vi "Get Data.vi"(8 "error in":errorcluster, 11 "3022A in":refnum<class "3022A.lvclass">) -> (0 "error out":errorcluster, 2 "DataOut":refnum<class "Data.lvclass">[](array[class]), 3 "3022A out":refnum<class "3022A.lvclass">)   [LabVIEW 2014, in "3022A.lvclass"]
doc: "Send a command to get the concentration. The index will indicate which concentration to retrieve, the default being the FP concentration."
uses:
  3022A.lvclass
  Controls/3022A/Enum Cmd.ctl
  reusable/Data/Array Data/Single 1-D/Single_Array.lvclass
  reusable/Data/Data.lvclass
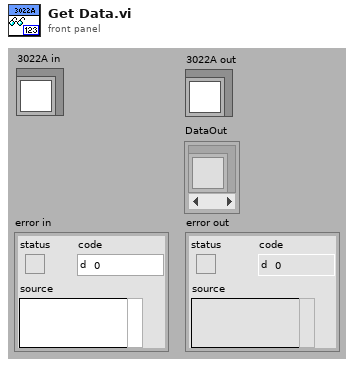
[diagram p1: front panel]
types:
  T1 = typedef "3022A.lvclass/Enum Cmd.ctl" = enum8{"CALIBRATE", "GET CAL DATA", "DUMP", "ESCAPE", "ID CAL LABEL", "INPUT CAL LABEL", "LIQUID LEVEL", "CONDENSER T", "SATURATOR T", "OPTICS T", "GET FLOW RATE", "READ ENV", "READ REF DETECTOR", "READ DETECTOR V", "READ 200 s BUFFER", "READ 20 s BUFFER", "READ 2 s BUFFER", "READ 1 s BUFFER", "READ PHOTOMETRIC CONC", "READ FP CONC", "READ MICROPROCESSOR PUMP CTL", "SENSOR", "SET VOLTAGE", "WRITE DISP MSG", "LASER OFF", "LASER ON", "PUMP OFF", "PUMP ON", "DRAIN", "FILL", "RESET CONC BUFFERS", "LOW FLOW MODE", "HIGH FLOW MODE"}
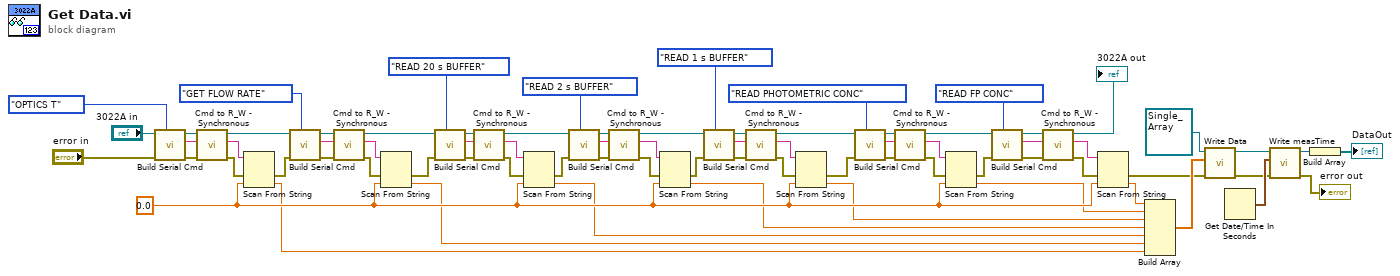
[diagram p0: block diagram]
diagram:
  w8 = sgl 0.0 ("default value 1")
  n1 = call-dynamic "Build Serial Cmd.vi"("Cmd"=Enum_Cmd."OPTICS T", "error in (no error)"="error in", "3022A in"="3022A in") -> ("error out"=w69:errorcluster, "Cmd Out"=w71:string, "3022A out"=w70:refnum<class "3022A.lvclass">)  [unwired: 6 in]
  n2 = call-dynamic "Cmd to R_W - Synchronous.vi"("error in"=w69, "write buffer"=w71, "Serial IO in"=w70) -> ("error out"=w68:errorcluster, "read buffer"=w67:string, "Serial IO out"=w56:refnum<class "3022A.lvclass">)  [unwired: 6 in]
  n3 = Scan From String(input string=w67, error in=w68, default 1=w8) -> (error out=w55:errorcluster, output 1=w7:sgl)  [unwired: 2 in, 2 out]
  n4 = call-dynamic "Build Serial Cmd.vi"("Cmd"=Enum_Cmd."GET FLOW RATE", "error in (no error)"=w55, "3022A in"=w56) -> ("error out"=w60:errorcluster, "Cmd Out"=w58:string, "3022A out"=w59:refnum<class "3022A.lvclass">)  [unwired: 6 in]
  n5 = call-dynamic "Cmd to R_W - Synchronous.vi"("error in"=w60, "write buffer"=w58, "Serial IO in"=w59) -> ("error out"=w61:errorcluster, "read buffer"=w62:string, "Serial IO out"=w42:refnum<class "3022A.lvclass">)  [unwired: 6 in]
  n6 = Scan From String(input string=w62, error in=w61, default 1=w8) -> (error out=w22:errorcluster, output 1=w6:sgl)  [unwired: 2 in, 2 out]
  n7 = call-dynamic "Build Serial Cmd.vi"("Cmd"=Enum_Cmd."READ 20 s BUFFER", "error in (no error)"=w22, "3022A in"=w42) -> ("error out"=w21:errorcluster, "Cmd Out"=w50:string, "3022A out"=w49:refnum<class "3022A.lvclass">)  [unwired: 6 in]
  n8 = call-dynamic "Cmd to R_W - Synchronous.vi"("error in"=w21, "write buffer"=w50, "Serial IO in"=w49) -> ("error out"=w20:errorcluster, "read buffer"=w47:string, "Serial IO out"=w41:refnum<class "3022A.lvclass">)  [unwired: 6 in]
  n9 = Scan From String(input string=w47, error in=w20, default 1=w8) -> (error out=w19:errorcluster, output 1=w5:sgl)  [unwired: 2 in, 2 out]
  n10 = call-dynamic "Build Serial Cmd.vi"("Cmd"=Enum_Cmd."READ 2 s BUFFER", "error in (no error)"=w19, "3022A in"=w41) -> ("error out"=w40:errorcluster, "Cmd Out"=w43:string, "3022A out"=w44:refnum<class "3022A.lvclass">)  [unwired: 6 in]
  n11 = call-dynamic "Cmd to R_W - Synchronous.vi"("error in"=w40, "write buffer"=w43, "Serial IO in"=w44) -> ("error out"=w39:errorcluster, "read buffer"=w46:string, "Serial IO out"=w32:refnum<class "3022A.lvclass">)  [unwired: 6 in]
  n12 = Scan From String(input string=w46, error in=w39, default 1=w8) -> (error out=w31:errorcluster, output 1=w4:sgl)  [unwired: 2 in, 2 out]
  n13 = call-dynamic "Build Serial Cmd.vi"("Cmd"=Enum_Cmd."READ 1 s BUFFER", "error in (no error)"=w31, "3022A in"=w32) -> ("error out"=w37:errorcluster, "Cmd Out"=w36:string, "3022A out"=w35:refnum<class "3022A.lvclass">)  [unwired: 6 in]
  n14 = call-dynamic "Cmd to R_W - Synchronous.vi"("error in"=w37, "write buffer"=w36, "Serial IO in"=w35) -> ("error out"=w38:errorcluster, "read buffer"=w33:string, "Serial IO out"=w25:refnum<class "3022A.lvclass">)  [unwired: 6 in]
  n15 = Scan From String(input string=w33, error in=w38, default 1=w8) -> (error out=w24:errorcluster, output 1=w3:sgl)  [unwired: 2 in, 2 out]
  n16 = call-dynamic "Build Serial Cmd.vi"("Cmd"=Enum_Cmd."READ PHOTOMETRIC CONC", "error in (no error)"=w24, "3022A in"=w25) -> ("error out"=w27:errorcluster, "Cmd Out"=w28:string, "3022A out"=w29:refnum<class "3022A.lvclass">)  [unwired: 6 in]
  n17 = call-dynamic "Cmd to R_W - Synchronous.vi"("error in"=w27, "write buffer"=w28, "Serial IO in"=w29) -> ("error out"=w26:errorcluster, "read buffer"=w30:string, "Serial IO out"=w12:refnum<class "3022A.lvclass">)  [unwired: 6 in]
  n18 = Scan From String(input string=w30, error in=w26, default 1=w8) -> (error out=w11:errorcluster, output 1=w2:sgl)  [unwired: 2 in, 2 out]
  n19 = call-dynamic "Build Serial Cmd.vi"("Cmd"=Enum_Cmd."READ FP CONC", "error in (no error)"=w11, "3022A in"=w12) -> ("error out"=w16:errorcluster, "Cmd Out"=w15:string, "3022A out"=w14:refnum<class "3022A.lvclass">)  [unwired: 6 in]
  n20 = call-dynamic "Cmd to R_W - Synchronous.vi"("error in"=w16, "write buffer"=w15, "Serial IO in"=w14) -> ("error out"=w17:errorcluster, "read buffer"=w13:string, "Serial IO out"=→"3022A out":refnum<class "3022A.lvclass">)  [unwired: 6 in]
  n21 = Scan From String(input string=w13, error in=w17, default 1=w8) -> (error out=w10:errorcluster, output 1=w1:sgl)  [unwired: 2 in, 2 out]
  n22 = Build Array(w1, w2, w3, w4, w5, w6, w7) -> (w51:sgl[])
  n23 = call "Write Data.vi"("error in (no error)"=w10, "Data"=w51, "Single_Array in"=refnum<class "Single_Array.lvclass"> refnum ("Base Data Class.lvlib:Single_Array.lvclass")) -> ("error out"=w52:errorcluster, "Single_Array out"=w53:refnum<class "Single_Array.lvclass">)  [unwired: 7 in]
  n24 = Get Date/Time In Seconds() -> (seconds since 1Jan1904=w66:timestamp)
  n25 = call "Write measTime.vi"("error in (no error)"=w52, "measTime"=w66, "Data in"=w53) -> ("error out"=→"error out":errorcluster, "Data out"=w64:refnum<class "Single_Array.lvclass">)  [unwired: 7 in]
  n26 = Build Array(w64) -> (→"DataOut":refnum<class "Single_Array.lvclass">[])
